vi "RESP3 data type attribute.vi"() -> (2 "dt attribute":string="_dt")   [LabVIEW 2019, in "RESP3.lvlib"]
uses:
  RESP3.lvlib
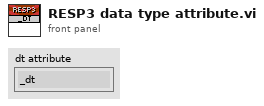
[diagram p1: front panel]
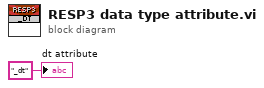
[diagram p0: block diagram]
diagram:
  "dt attribute" <- "_dt"
